vi "Pin PWM.vi"() -> ()   [LabVIEW 2014, in "STM32F4 Discovery General Wrapper.lvlib"]
uses:
  <vilib>/Aledyne-TSXperts/Arduino Compatible Compiler for LabVIEW/addons/STM32F4 Discovery General Wrapper/STM32F4 Discovery General Wrapper.lvlib
  <vilib>/Aledyne-TSXperts/Arduino Compatible Compiler for LabVIEW/addons/STM32F4 Discovery General Wrapper/Ctl/PinList.ctl
  <vilib>/Aledyne-TSXperts/Arduino Compatible Compiler for LabVIEW/addons/STM32F4 Discovery General Wrapper/Ctl/PinModes.ctl
  <vilib>/Aledyne-TSXperts/Arduino Compatible Compiler for LabVIEW/Arduino Compatible Compiler for LabVIEW.lvlib
  <vilib>/Aledyne-TSXperts/Arduino Compatible Compiler for LabVIEW/Code Generator/Arduino APIs/Digital/PinDirection.ctl
panel:
  out "error out":errorcluster
  in  "error in (no error)":errorcluster
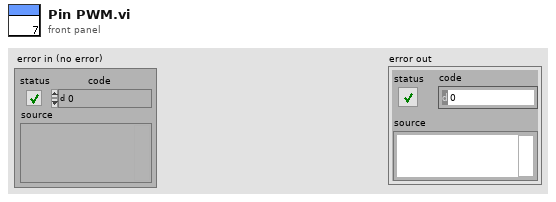
[diagram p1: front panel]
types:
  T1 = typedef "STM32F4 Discovery General Wrapper.lvlib/PinList.ctl" = enum8{"PA0", "PA1", "PA2", "PA3", "PA4", "PA5", "PA6", "PA7", "PA8", "PA9", "PA10", "PA11", "PA12", "PA13", "PA14", "PA15", "PB0", "PB1", "PB2", "PB3", "PB4", "PB5", "PB6", "PB7", "PB8", "PB9", "PB10", "PB11", "PB12", "PB13", "PB14", "PB15", "PC0", "PC1", "PC2", "PC3", "PC4", "PC5", "PC6", "PC7", "PC8", "PC9", "PC10", "PC11", "PC12", "PC13", "PC14", "PC15", "PD0", "PD1", "PD2", "PD3", "PD4", "PD5", "PD6", "PD7", "PD8", "PD9", "PD10", "PD11", "PD12", "PD13", "PD14", "PD15", "PE0", "PE1", "PE2", "PE3", "PE4", "PE5", "PE6", "PE7", "PE8", "PE9", "PE10", "PE11", "PE12", "PE13", "PE14", "PE15", "PF0", "PF1", "PF2", "PF3", "PF4", "PF5", "PF6", "PF7", "PF8", "PF9", "PF10", "PF11", "PF12", "PF13", "PF14", "PF15", "PG0", "PG1", "PG2", "PG3", "PG4", "PG5", "PG6", "PG7", "PG8", "PG9", "PG10", "PG11", "PG12", "PG13", "PG14", "PG15"}
  T2 = typedef "Arduino Compatible Compiler for LabVIEW.lvlib/PinDirection.ctl" = enum16{" INPUT", "OUTPUT", " INPUT_PULLUP"}
  T3 = typedef "STM32F4 Discovery General Wrapper.lvlib/PinModes.ctl" = enum16{"OUTPUT", "OUTPUT_OPEN_DRAIN", "INPUT", "INPUT_ANALOG", "INPUT_PULLUP", "INPUT_PULLDOWN", "INPUT_FLOATING", "PWM", "PWM_OPEN_DRAIN"}
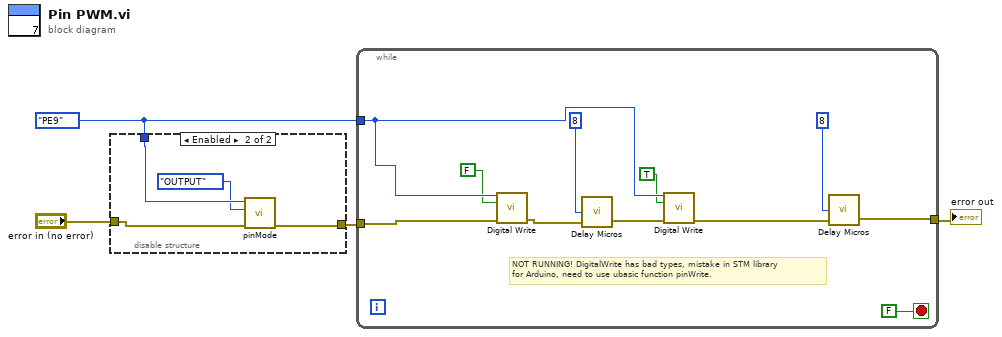
[diagram p0: block diagram]
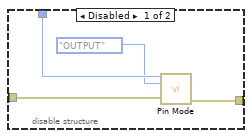
[diagram p2: hidden frame]
diagram:
  w1 = PinList."PE9" ("Pin number")
  n1 = disable-structure shown="Enabled" {
    disable-tunnel: [w8 w11] -> w4
    disable-tunnel: "error in (no error)" -> [w7 w12]
    disable-tunnel: w1 -> [w6 w10]
    frame Disabled {
      n2 = call <vilib>:"Pin Mode.vi"("pin"=w6, "direction"=PinDirection."OUTPUT", "error in (no error)"=w7) -> ("error out"=w8:errorcluster)  [unwired: 12 in]
    }
    frame Enabled {
      n3 = call <vilib>:"pinMode.vi"("Error In"=w12, "Pin mode"=PinModes."OUTPUT", "Pin number"=w10) -> ("Error Out"=w11:errorcluster)  [unwired: 8 in]
    }
  }
  n4 = while {
    tunnel: w1 -> [w15]
    tunnel: [w21] -> w2
    tunnel: w4 -> [w17]
    stop <- FALSE stop-if-true
    # "NOT RUNNING! DigitalWrite has bad types, mistake in STM library\nfor Arduino, need to use ubasic function pinWrite."
    n5 = call <vilib>:"Digital Write.vi"("pin"=w15, "state"=FALSE, "error in (no error)"=w17) -> ("error out"=w18:errorcluster)  [unwired: 12 in]
    n6 = call <vilib>:"Delay Micros.vi"("error in (no error)"=w18, "delay"=u16 8) -> ("error out"=w19:errorcluster)  [unwired: 2 in]
    n7 = call <vilib>:"Digital Write.vi"("pin"=w15, "state"=TRUE, "error in (no error)"=w19) -> ("error out"=w20:errorcluster)  [unwired: 12 in]
    n8 = call <vilib>:"Delay Micros.vi"("error in (no error)"=w20, "delay"=u16 8) -> ("error out"=w21:errorcluster)  [unwired: 2 in]
  }
  "error out" <- w2
